vi "Timeout triggered.vi"(9 "Timeout (ms)":u32, 11 "Initial Timer Value":u32) -> (2 "Triggered":bool)   [LabVIEW 2017, in "SSH.lvlib"]
doc: "Analyses the tick count to determine if a timeout has been triggered"
uses:
  SSH.lvlib
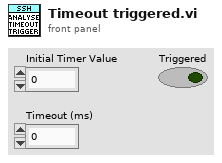
[diagram p1: front panel]
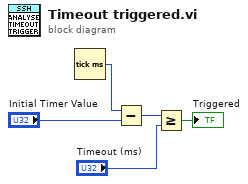
[diagram p0: block diagram]
diagram:
  n1 = Tick Count (ms)() -> (millisecond timer value=w1:u32)
  n2 = Subtract(x=w1, y="Initial Timer Value") -> (x-y=w2:u32)
  n3 = Greater Or Equal?(x=w2, y="Timeout (ms)") -> (x >= y?=→"Triggered":bool)
